vi "get freq correction.vi"(8 "error in (no error)":errorcluster, 11 "DeviceRefnum":u64) -> (0 "error out":errorcluster, 2 "Frequency Correction":i32, 3 "DeviceRefnum Out":u64)   [LabVIEW 2015, in "rtlsdr.lvlib"]
doc: "Get actual frequency correction value of the device."
uses:
  rtlsdr.lvlib
  rtlsdr/rtlsdr.dll
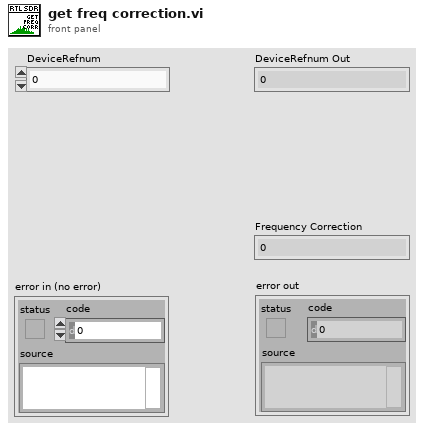
[diagram p1: front panel]
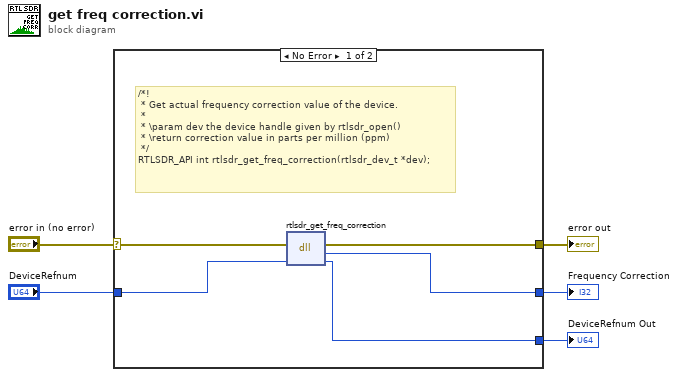
[diagram p0: block diagram]
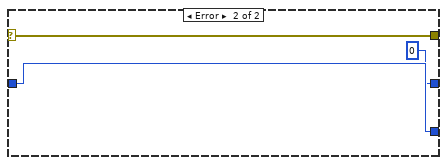
[diagram p2: hidden frame]
diagram:
  n1 = case shown="No Error" "error in (no error)" {
    selector: "error in (no error)" -> [w6 w13]
    tunnel: [w10 0 ("return type")] -> w5
    tunnel: [w9 w13] -> w4
    tunnel: "DeviceRefnum" -> [w8 w12]
    tunnel: [w7 w12] -> w2
    frame No Error {
      # "/*!\n * Get actual frequency correction value of the device.\n *\n * \\param dev the device handle given by rtlsdr_open()\n * \\return correction value in parts per million (ppm)\n */\nRTLSDR_API int rtlsdr_get_freq_correction(rtlsdr_dev_t *dev);"
      n2 = dll-call lib="C:/Users/TheDoctor/Documents/Projects/Labview Libraries/rtlsdr/rtlsdr.*" fn="rtlsdr_get_freq_correction"(error in=w6, "DeviceRefnum"=w8) -> (error out=w9:errorcluster, "return type"=w10:i32, "DeviceRefnum"=w7:u64)  [unwired: 2 in, 1 out]
    }
    frame Error {
    }
  }
  "Frequency Correction" <- w5
  "error out" <- w4
  "DeviceRefnum Out" <- w2
